vi "Configure L3G4200D.vi"(8 "error in":errorcluster, 11 "FPGA VI Reference":T1) -> (0 "error out":errorcluster, 3 "FPGA VI Reference Out":T1)   [LabVIEW 2014]
uses:
  Controls/FPGA Reference.ctl
  Controls/SPI Configuration Cluster.ctl
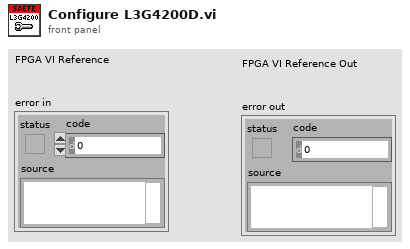
[diagram p1: front panel]
types:
  T1 = typedef "FPGA Reference.ctl" = refnum<k20>
  T2 = typedef "SPI Configuration Cluster.ctl" = cluster{"CS":u8, "Clock Rate (Hz)":dbl, "Clock Mode":u8, "CS Active State":bool}
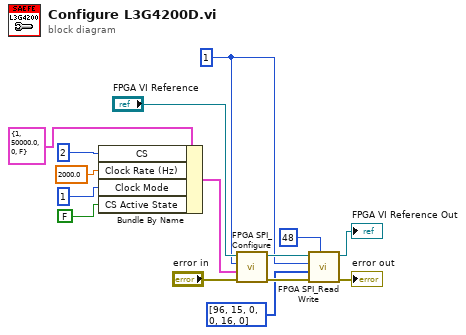
[diagram p0: block diagram]
diagram:
  w5 = i8 1 ("Port")
  n1 = Bundle By Name(cluster=T2 {"CS"=1, "Clock Rate (Hz)"=50000.0, "Clock Mode"=0, "CS Active State"=FALSE} ("Configuration Cluster"), "CS"=u8 2, "Clock Rate (Hz)"=2000.0, "Clock Mode"=u8 1, "CS Active State"=FALSE) -> (w12:T2)
  n2 = call "FPGA SPI_Configure.vi"("error in"="error in", "Configuration Cluster"=w12, "Port"=w5, "FPGA VI Reference"="FPGA VI Reference") -> ("error out"=w6:errorcluster, "FPGA VI Reference Out"=w7:T1)  [unwired: 5 in, 1 out]
  n3 = call "FPGA SPI_Read Write.vi"("Total Bits"=u16 48, "error in"=w6, "Write Data"=u8[] [96, 15, 0, 0, 16, 0], "Port"=w5, "FPGA VI Reference"=w7) -> ("error out"=→"error out":errorcluster, "FPGA VI Reference Out"=→"FPGA VI Reference Out":T1)  [unwired: 4 in, 1 out]
